vi "Configure Voltage.vi"(8 "error in (no error)":errorcluster, 10 "Voltage":dbl, 11 "Power Supply in":refnum<class "Power Supply.lvclass">) -> (0 "error out":errorcluster, 3 "Power Supply out":refnum<class "Power Supply.lvclass">)   [LabVIEW 2020, in "Power Supply.lvclass"]
uses:
  Power Supply.lvclass
  Power Supply.lvclass/Power Supply.ctl
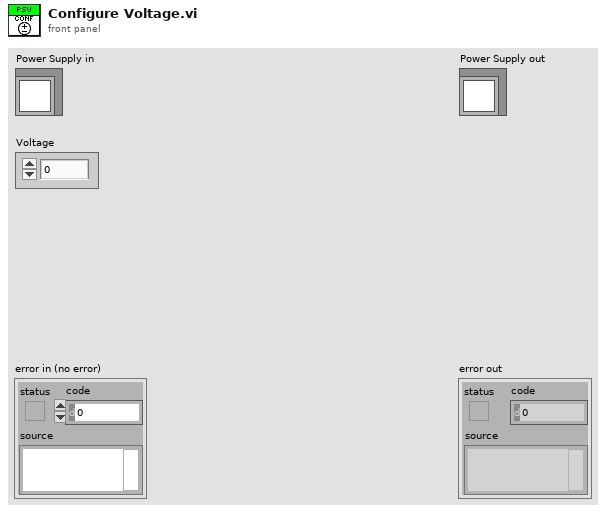
[diagram p1: front panel]
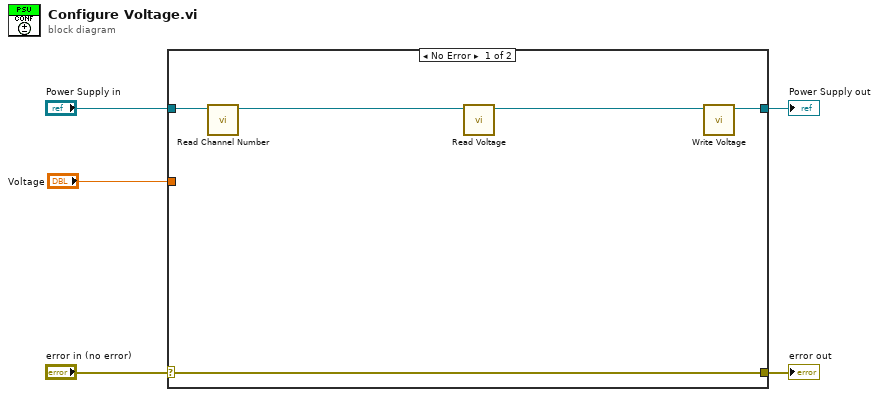
[diagram p0: block diagram]
diagram:
  n1 = case shown="No Error" "error in (no error)" {
    selector: "error in (no error)" -> [w10 w12]
    tunnel: [w10 w12] -> w4
    tunnel: [w8 w11] -> w2
    tunnel: "Power Supply in" -> [w7 w11]
    tunnel: "Voltage" -> [_ _]
    frame No Error {
      n2 = call "Read Channel Number.vi"("Power Supply in"=w7) -> ("Power Supply out"=w6:refnum<class "Power Supply.lvclass">)  [unwired: 9 in, 1 out]
      n3 = call "Read Voltage.vi"("Power Supply in"=w6) -> ("Power Supply out"=w9:refnum<class "Power Supply.lvclass">)  [unwired: 9 in, 1 out]
      n4 = call "Write Voltage.vi"("Power Supply in"=w9) -> ("Power Supply out"=w8:refnum<class "Power Supply.lvclass">)  [unwired: 10 in]
    }
    frame Error {
    }
  }
  "error out" <- w4
  "Power Supply out" <- w2
